vi "2700读取电压.vi"(8 "error in (no error)":errorcluster, 11 "VISA resource name":refnum<visa-resource-name>="GPIB0::16::INSTR") -> (0 "error out":errorcluster, 3 "VISA resource name out":refnum<visa-resource-name>)   [LabVIEW 2021]
uses:
  <instrlib>/Keithley 27XX/Keithley 27XX.lvlib
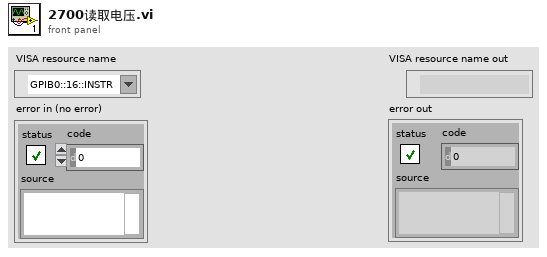
[diagram p1: front panel]
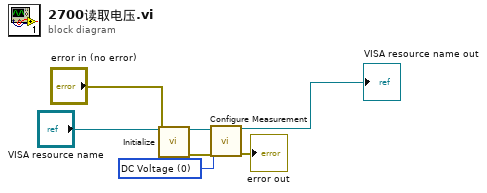
[diagram p0: block diagram]
diagram:
  w5 = u16 0 items=["DC Voltage", "AC Voltage", "DC Current", "AC Current", "Resistance", "Four-Wire Resistance", "Temperature", "Frequency", "Period", "Continuity"] ("Function (0: DC Voltage)")
  n1 = call <instrlib>:"Initialize.vi"("VISA resource name"="VISA resource name", "error in (no error)"="error in (no error)") -> ("VISA resource name out"=w7:refnum<visa-resource-name>, "error out"=w6:errorcluster)  [unwired: 12 in]
  n2 = call <instrlib>:"Configure Measurement.vi"("VISA resource name"=w7, "Function (0: DC Voltage)"=w5, "error in (no error)"=w6) -> ("VISA resource name out"=→"VISA resource name out":refnum<visa-resource-name>, "error out"=→"error out":errorcluster)  [unwired: 11 in]
